vi "Error_1.vi"(7 "PNGs in folder":string[](array[string]), 8 "error in (no error)":errorcluster) -> (0 "error out":errorcluster)   [LabVIEW 2023]
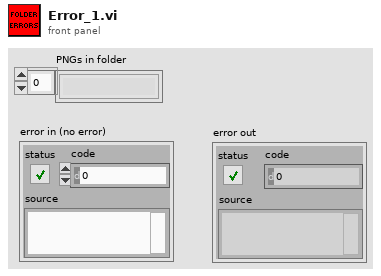
[diagram p1: front panel]
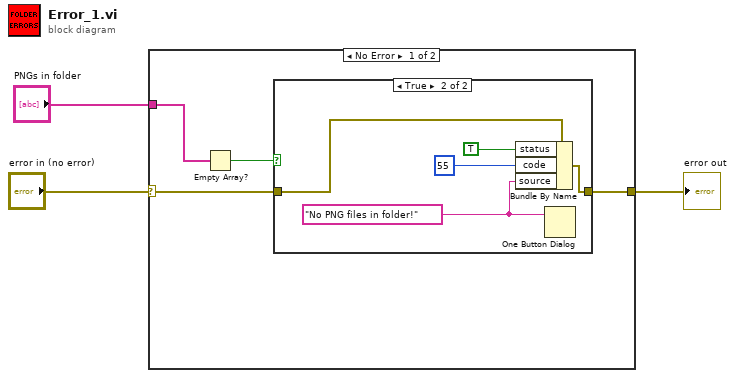
[diagram p0: block diagram]
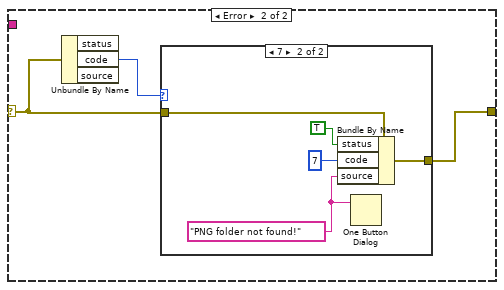
[diagram p3: hidden frame]
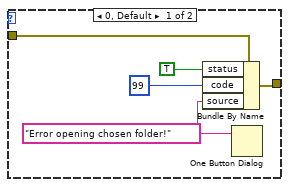
[diagram p4: hidden frame]
diagram:
  n1 = case shown="No Error" "error in (no error)" {
    selector: "error in (no error)" -> [w5 w15]
    tunnel: "PNGs in folder" -> [w7 _]
    tunnel: [w4 w14] -> w1
    frame No Error {
      n2 = Empty Array?(array=w7) -> (empty?=w6:bool)
      n3 = case shown="True" w6 {
        tunnel: w5 -> [w8 w12]
        tunnel: [w8 w9] -> w4
        frame False {
        }
        frame True {
          w10 = "No PNG files in folder!"
          n4 = Bundle By Name(cluster=w12, "status"=TRUE ("status\nstatus"), "code"=55, "source"=w10) -> (w9:errorcluster)
          n5 = One Button Dialog(message=w10) -> ()  [unwired: 1 in, 1 out]
        }
      }
    }
    frame Error {
      n6 = Unbundle By Name(w15) -> ("code"=w16:i32)  [unwired: 2 out]
      n7 = case shown="7" w16 {
        tunnel: w15 -> [w21 w26]
        tunnel: [w17 w23] -> w14
        frame 0, Default {
          w18 = "Error opening chosen folder!"
          n8 = Bundle By Name(cluster=w21, "status"=TRUE, "code"=99, "source"=w18) -> (w17:errorcluster)
          n9 = One Button Dialog(message=w18) -> ()  [unwired: 1 in, 1 out]
        }
        frame 7 {
          w22 = "PNG folder not found!"
          n10 = Bundle By Name(cluster=w26, "status"=TRUE, "code"=7, "source"=w22) -> (w23:errorcluster)
          n11 = One Button Dialog(message=w22) -> ()  [unwired: 1 in, 1 out]
        }
      }
    }
  }
  "error out" <- w1
